vi "Generated Descriptors.vi"() -> (3 "Descriptor Strings":string[](array[string]))   [LabVIEW 2021, in "streamtest_server.lvlib"]
uses:
  streamtest_server.lvlib
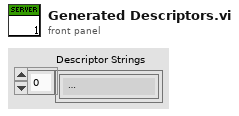
[diagram p1: front panel]
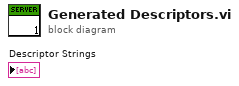
[diagram p0: block diagram]
diagram:
